vi "Holo Position.vi"(0 "Notifier Name":string, 7 "Holo Position":i32[](array[numeric]), 11 "Error In":errorcluster) -> (4 "Notifier Name Dup":string, 8 "SLM Status":T1, 15 "Error Out":errorcluster)   [LabVIEW 2018]
uses:
  Hamamatsu/X10468 Series/X10468 Controls/X10468 SLM Notifier.ctl
  Hamamatsu/X10468 Series/X10468 Controls/X10468 SLM Actions.ctl
  <vilib>/vision/Image Controls.llb/IMAQ Image.ctl
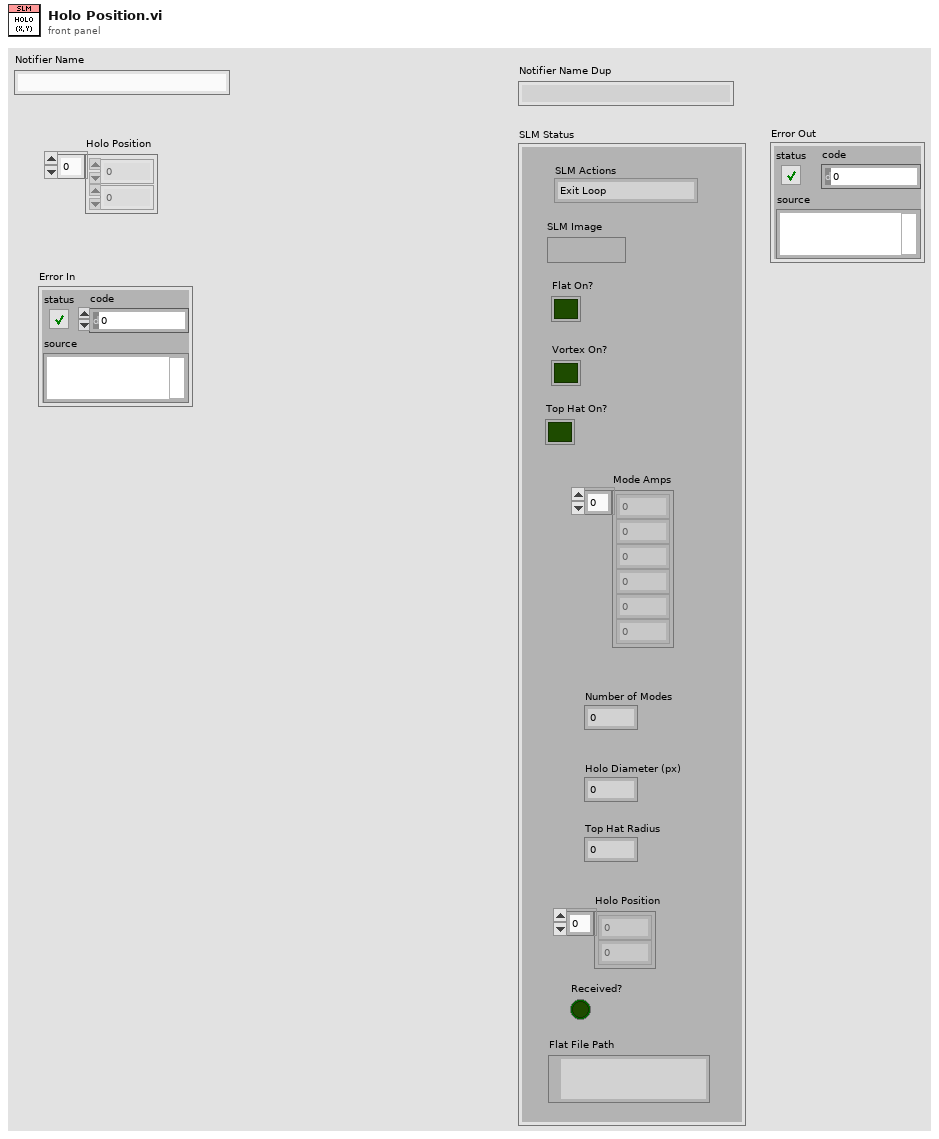
[diagram p1: front panel]
types:
  T1 = typedef "X10468 SLM Notifier.ctl" = cluster{"SLM Actions":T2, "SLM Image":T3, "Flat On?":bool, "Vortex On?":bool, "Top Hat On?":bool, "Mode Amps":dbl[], "Number of Modes":i32, "Holo Diameter (px)":i32, "Top Hat Radius":dbl, "Holo Position":i32[], "Received?":bool, "Flat File Path":path}
  T2 = typedef "X10468 SLM Actions.ctl" = enum16{"Exit Loop", "Get Settings", "Set Flat File", "Change Holo Size", "Change Num Modes", "Change Holo Position", "Change Top Hat Size", "Change Vortex Direction", "Change Mode Amounts", "Flat On/Off", "Vortex On/Off", "Top Hat On/Off", "Make Hologram", "Update SLM Display", "Quit"}
  T3 = typedef "IMAQ Image.ctl" = refnum<image>
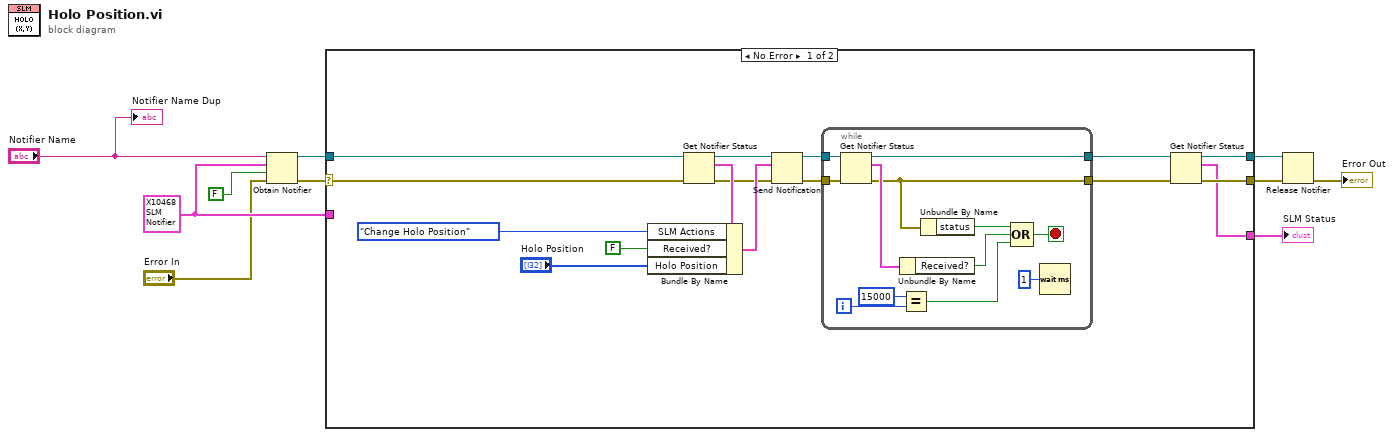
[diagram p0: block diagram]
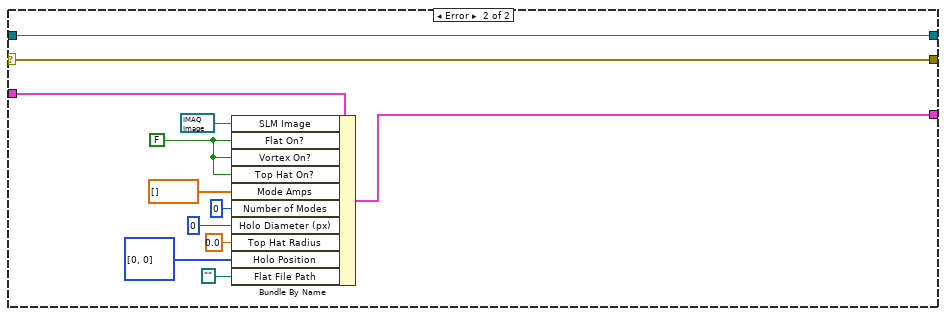
[diagram p2: hidden frame]
diagram:
  w2 = T1 {"SLM Actions"=enum."Exit Loop", "SLM Image"=refnum, "Flat On?"=FALSE, "Vortex On?"=FALSE, "Top Hat On?"=FALSE, "Mode Amps"=[], "Number of Modes"=0, "Holo Diameter (px)"=0, "Top Hat Radius"=0.0, "Holo Position"=[], "Received?"=FALSE, "Flat File Path"=path ""} ("SLM Notifier")
  n1 = Obtain Notifier(name (unnamed)="Notifier Name", notification data type=w2, create if not found? (T)=FALSE, error in (no error)="Error In") -> (notifier out=w8:refnum<notifier>, error out=w7:errorcluster)  [unwired: 1 out]
  n2 = case shown="No Error" w7 {
    selector: w7 -> [w24 w49]
    tunnel: w8 -> [w25 w50]
    tunnel: [w21 w50] -> w6
    tunnel: [w20 w49] -> w5
    tunnel: [w19 w47] -> w3
    tunnel: w2 -> [_ w48]
    frame No Error {
      n3 = Get Notifier Status(notifier=w25, error in (no error)=w24) -> (notifier out=w18:refnum<notifier>, current notification=w17:T1, error out=w15:errorcluster)  [unwired: 2 out]
      n4 = Bundle By Name(cluster=w17, "SLM Actions"=X10468_SLM_Actions."Change Holo Position", "Received?"=FALSE, "Holo Position"="Holo Position") -> (w16:T1)
      n5 = Send Notification(notification=w16, notifier=w18, error in (no error)=w15) -> (notifier out=w13:refnum<notifier>, error out=w12:errorcluster)
      n6 = while {
        tunnel: w13 -> [w38]
        tunnel: [w35] -> w23
        tunnel: w12 -> [w32]
        tunnel: [w31] -> w22
        i -> [w34]
        stop <- w27 stop-if-true
        n7 = Get Notifier Status(notifier=w38, error in (no error)=w32) -> (notifier out=w35:refnum<notifier>, current notification=w37:T1, error out=w31:errorcluster)  [unwired: 2 out]
        n8 = Unbundle By Name(w37) -> ("Received?"=w29:bool)
        n9 = Equal?(x=15000, y=w34) -> (x = y?=w28:bool)
        n10 = Unbundle By Name(w31) -> ("status"=w30:bool)
        n11 = Compound Arithmetic op=OR(w30, w29, w28) -> (w27:bool)
        n12 = Wait (ms)(milliseconds to wait=u32 1) -> ()  [unwired: 1 out]
      }
      n13 = Get Notifier Status(notifier=w23, error in (no error)=w22) -> (notifier out=w21:refnum<notifier>, current notification=w19:T1, error out=w20:errorcluster)  [unwired: 2 out]
    }
    frame Error {
      w45 = FALSE ("Flat On?")
      n14 = Bundle By Name(cluster=w48, "SLM Image"=T3 refnum, "Flat On?"=w45, "Vortex On?"=w45, "Top Hat On?"=w45, "Mode Amps"=dbl[] [], "Number of Modes"=0, "Holo Diameter (px)"=0, "Top Hat Radius"=0.0, "Holo Position"=i32[] [0, 0], "Flat File Path"=path "") -> (w47:T1)
    }
  }
  "SLM Status" <- w3
  n15 = Release Notifier(notifier=w6, error in (no error)=w5) -> (error out=→"Error Out":errorcluster)  [unwired: 1 in, 2 out]
  "Notifier Name Dup" <- "Notifier Name"
